vi "SetAngleSetpoint.vi"(8 "error in (no error)":errorcluster, 10 "angleSetpointInput":dbl, 11 "DriveBase.lvclass":refnum<class "DriveBase.lvclass">) -> (0 "error out":errorcluster, 3 "DriveBase.lvclass":refnum<class "DriveBase.lvclass">)   [LabVIEW 2016, in "DriveBase.lvclass"]
uses:
  DriveBase.lvclass
  DriveBase.lvclass/DriveBase.ctl
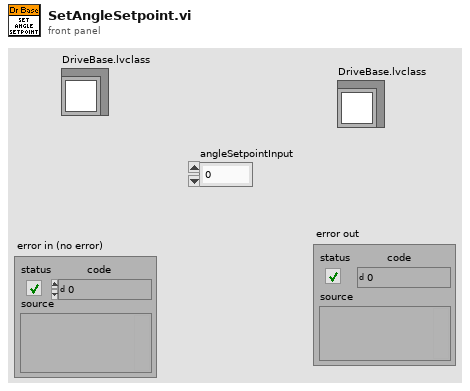
[diagram p1: front panel]
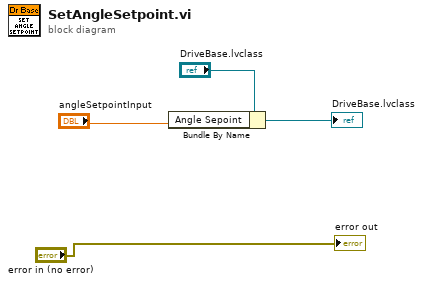
[diagram p0: block diagram]
diagram:
  n1 = Bundle By Name(cluster="DriveBase.lvclass", "Angle Sepoint"="angleSetpointInput") -> (→"DriveBase.lvclass":refnum<class "DriveBase.lvclass">)
  "error out" <- "error in (no error)"
